vi "N5.vi"() -> ()   [LabVIEW 2020]
uses:
  <vilib>/numeric/Random Number (Range) U64.vi
  <vilib>/numeric/sub_Random U32.vi
panel:
  out "Second max value":u64
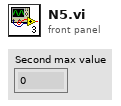
[diagram p1: front panel]
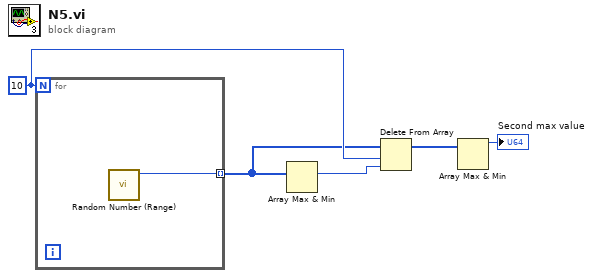
[diagram p0: block diagram]
diagram:
  w4 = 10
  n1 = for {
    N: w4 -> [_]
    tunnel: [w6] -> w3 mode=indexing
    n2 = call-poly <vilib>:"Random Number (Range).vi"() -> ("number"=w6:u64)  [unwired: 11 in]
  }
  n3 = Array Max & Min(array=w3) -> (max index (indices)=w5:i32)  [unwired: 3 out]
  n4 = Delete From Array(array=w3, length=w4, index=w5) -> (array with subset deleted=w2:u64[])  [unwired: 1 out]
  n5 = Array Max & Min(array=w2) -> (max value=→"Second max value":u64)  [unwired: 3 out]
